vi "Method.vi"(4 "Input B":refnum<class "Abs_Numeric.lvclass">, 5 "Input A":T1) -> (1 "Result":T1)   [LabVIEW 2021, in "Divide_CPLX_EXT.lvclass"]
uses:
  Divide_CPLX_EXT.lvclass
  Abs Type.ctl
  Abs_Types/Complex Extended Float/Complex Extended Float.lvclass
  Abs_Types/Numeric/Abs_Numeric.lvclass
  C:/Users/Tim/Documents/LabVIEW/2021/Data Classes/Source/Functions/Support/Two Terminal/Cmplx EXT/AbsFunc_Two Term_Complex EXT.lvclass
  C:/Users/Tim/Documents/LabVIEW/2021/Data Classes/Source/Abs_Types/Complex Extended Float/Complex Extended Float.lvclass
  Support/Two Terminal/Cmplx EXT/AbsFunc_Two Term_Complex EXT.lvclass/AbsFunc_Two Term_Complex EXT.ctl
  Support/Two Terminal/Cmplx EXT/Properties/Write Numeric A.vi
  Support/Two Terminal/Cmplx EXT/Properties/Write Numeric B.vi
  Divide_CPLX_EXT.lvclass/Divide_CPLX_EXT.ctl
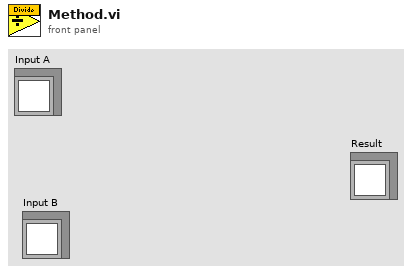
[diagram p1: front panel]
types:
  T1 = typedef "Divide_CPLX_EXT.lvclass/Abs Type.ctl" = refnum<class "Complex Extended Float.lvclass">
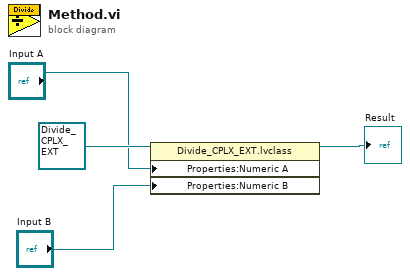
[diagram p0: block diagram]
diagram:
  n1 = property class="Divide_CPLX_EXT.lvclass"(reference=refnum<class "Divide_CPLX_EXT.lvclass"> refnum ("Functions.lvlib:Numeric.lvlib:Divide.lvclass"), "Properties:Numeric A"="Input A", "Properties:Numeric B"="Input B") -> (reference out=→"Result":refnum<class "Divide_CPLX_EXT.lvclass">)  [unwired: 1 in, 1 out]
